vi "Format_Write.vi"(0 "Source Address":u32=15, 1 "Register 0 Write?":bool, 2 "Address":u32=31, 3 "Address Parity":u32=1, 5 "error in (no error)":errorcluster, 7 "Data":u32=255, 8 "CMD":u32=2, 9 "Data Parity":u32=1) -> (15 "RFFE Write Word":u32, 19 "error out":errorcluster)   [LabVIEW 2020, in "niDigital.lvclass"]
uses:
  niDigital.lvclass
panel:
  out "x << y 8":u32
  out "x << y 7":u32
  out "x << y 6":u32
  out "x << y 5":u32
  out "x << y 4":u32=512
  out "x << y 3":u32=15872
  out "x << y 2":u32=131072
  out "x << y":u32=491520
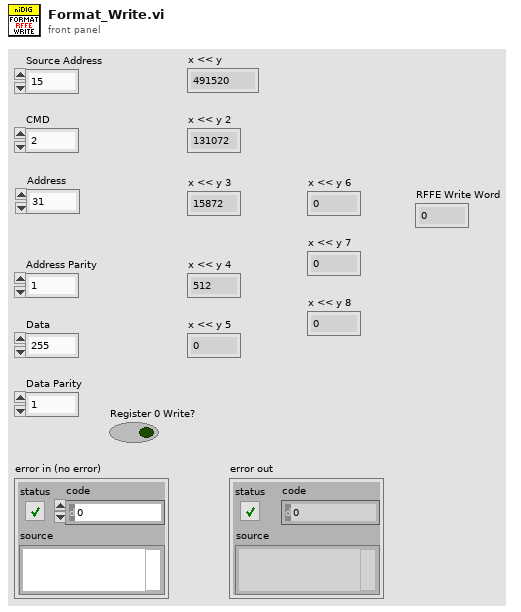
[diagram p1: front panel]
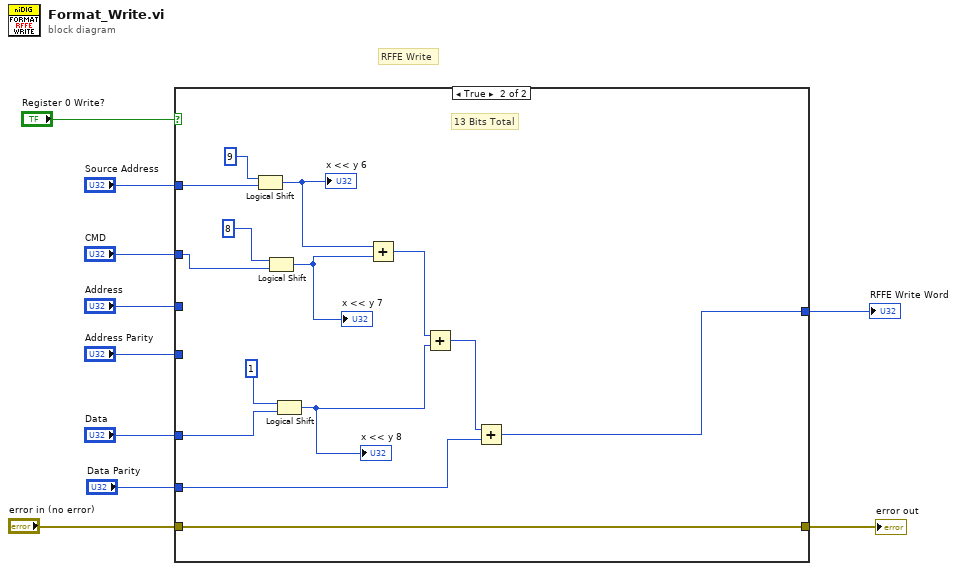
[diagram p0: block diagram]
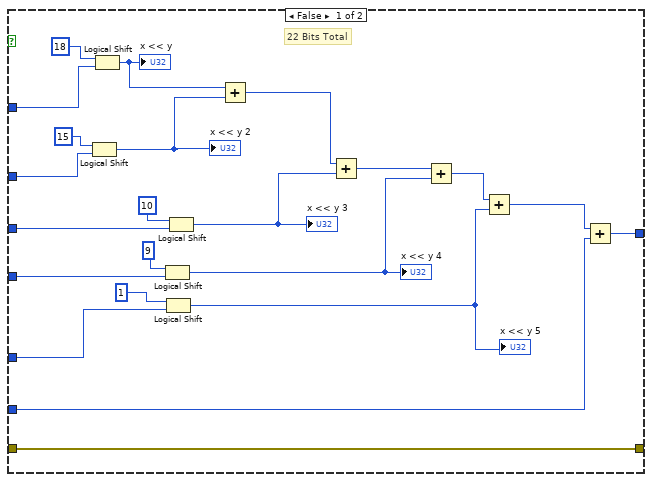
[diagram p2: hidden frame]
diagram:
  # "RFFE Write"
  n1 = case shown="True" "Register 0 Write?" {
    tunnel: "Source Address" -> [w32 w46]
    tunnel: "CMD" -> [w31 w36]
    tunnel: "Address" -> [w30 _]
    tunnel: "Address Parity" -> [w29 _]
    tunnel: "Data" -> [w28 w43]
    tunnel: "Data Parity" -> [w27 w38]
    tunnel: [w26 w37] -> w4
    tunnel: "error in (no error)" -> [w11 w33]
    tunnel: [w11 w33] -> w1
    frame False {
      # "22 Bits Total"
      n2 = Logical Shift(y=i16 15, x=w31) -> (x << y=w22:u32)
      "x << y 2" <- w22
      n3 = Logical Shift(y=i16 18, x=w32) -> (x << y=w24:u32)
      "x << y" <- w24
      n4 = Logical Shift(y=i16 9, x=w29) -> (x << y=w16:u32)
      "x << y 4" <- w16
      n5 = Logical Shift(y=i16 1, x=w28) -> (x << y=w13:u32)
      "x << y 5" <- w13
      n6 = Logical Shift(y=i16 10, x=w30) -> (x << y=w20:u32)
      "x << y 3" <- w20
      n7 = Add(x=w24, y=w22) -> (x+y=w21:u32)
      n8 = Add(x=w21, y=w20) -> (x+y=w17:u32)
      n9 = Add(x=w17, y=w16) -> (x+y=w14:u32)
      n10 = Add(x=w14, y=w13) -> (x+y=w12:u32)
      n11 = Add(x=w12, y=w27) -> (x+y=w26:u32)
    }
    frame True {
      # "13 Bits Total"
      n12 = Logical Shift(y=i16 9, x=w46) -> (x << y=w44:u32)
      "x << y 6" <- w44
      n13 = Logical Shift(y=i16 8, x=w36) -> (x << y=w34:u32)
      "x << y 7" <- w34
      n14 = Logical Shift(y=i16 1, x=w43) -> (x << y=w40:u32)
      "x << y 8" <- w40
      n15 = Add(x=w44, y=w34) -> (x+y=w41:u32)
      n16 = Add(x=w41, y=w40) -> (x+y=w39:u32)
      n17 = Add(x=w39, y=w38) -> (x+y=w37:u32)
    }
  }
  "RFFE Write Word" <- w4
  "error out" <- w1
